vi "RobotDataReturnTest.vi"() -> ()   [LabVIEW 2024]
panel:
  out "Array":dbl[](array[numeric])
  out "error out":errorcluster
  in  "ip":string
  in  "error in (no error)":errorcluster
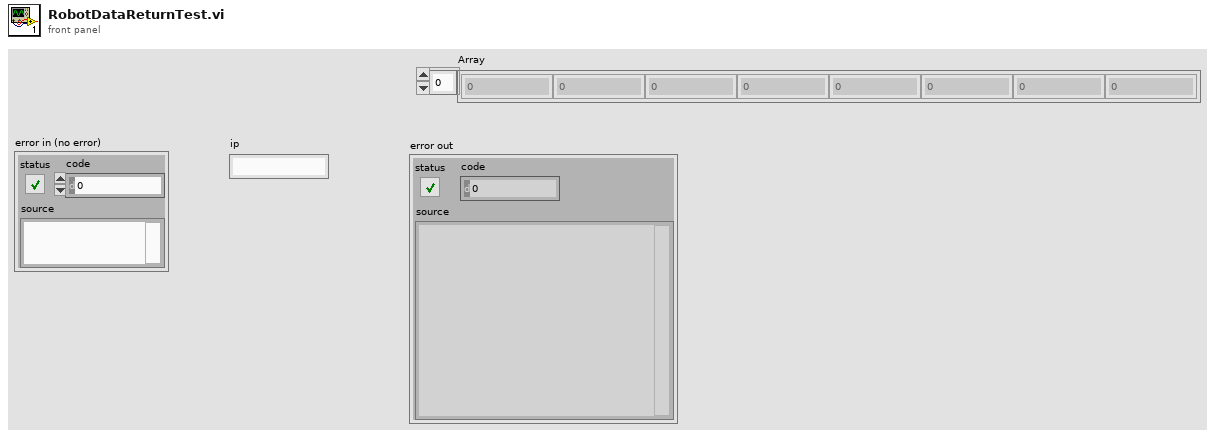
[diagram p1: front panel]
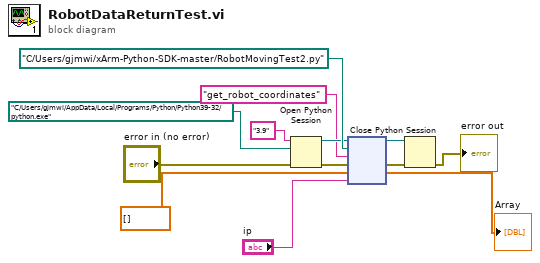
[diagram p0: block diagram]
diagram:
  n1 = Open Python Session(python version="3.9" ("Python version"), python path=path "C:/Users/gjmwi/AppData/Local/Programs/Python/Python39-32/python.exe" ("Python path"), 3:"error in (no error)") -> (session out=w9:refnum<k35>, error out=w8:errorcluster)
  n2 = node(w9, path "C:/Users/gjmwi/xArm-Python-SDK-master/RobotMovingTest2.py" ("module path"), "get_robot_coordinates" ("function name"), w8, dbl[] [], "ip") -> (w6:refnum<k35>, w5:errorcluster, →"Array":dbl[])  [unwired: 1 in, 2 out]
  n3 = Close Python Session(session in=w6, error in=w5) -> (11:→"error out":errorcluster)
